vi "write hi scores.vi"(8 "Error In":errorcluster, 10 "file path (dialog if empty)":path, 11 "Score Array In":T1[](array[typedef])) -> (0 "Error Out":errorcluster)   [LabVIEW 2017]
uses:
  controls/scores.ctl
  <vilib>/Utility/file.llb/Write To Spreadsheet File (DBL).vi
  <vilib>/Utility/file.llb/Write To Spreadsheet File (string).vi
panel:
  out "initialized array":string[](array[string])
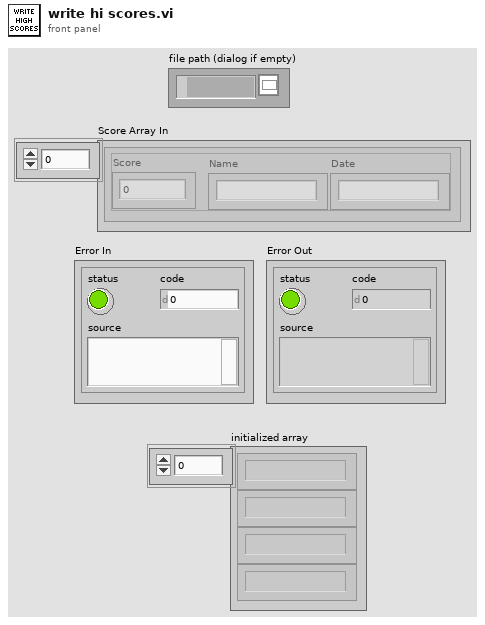
[diagram p1: front panel]
types:
  T1 = typedef "scores.ctl" = cluster{"Score":dbl, "Name":string, "Date":string}
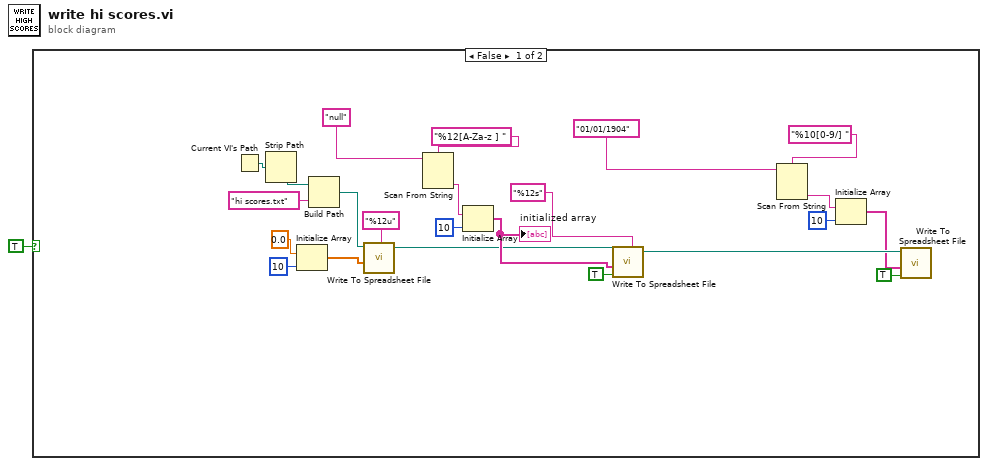
[diagram p0: block diagram]
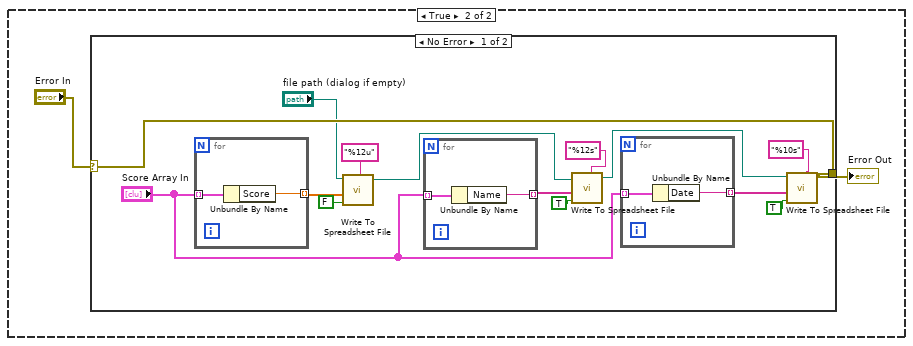
[diagram p2: hidden frame]
diagram:
  n1 = case shown="False" TRUE {
    frame False {
      n2 = Current VI's Path() -> (path=w13:path)
      n3 = Strip Path(path=w13) -> (stripped path=w12:path)  [unwired: 1 out]
      n4 = Initialize Array(0.0 ("element"), 10 ("dimension size")) -> (w15:dbl[])
      n5 = Build Path(base path=w12, name or relative path="hi scores.txt") -> (appended path=w16:path)
      n6 = call-poly <vilib>:"Write To Spreadsheet File.vi"("format (%.3f)"="%12u", "1D data"=w15, "file path (dialog if empty)"=w16) -> ("new file path (Not A Path if cancelled)"=w17:path)  [unwired: 5 in]
      n7 = Scan From String(format string="%12[A-Za-z ] ", input string="null") -> (output 1=w21:string)  [unwired: 3 in, 3 out]
      n8 = Initialize Array(w21, 10 ("dimension size")) -> (w24:string[])
      "initialized array" <- w24
      n9 = call-poly <vilib>:"Write To Spreadsheet File.vi"("format (%s)"="%12s" ("format (%12s)"), "append to file? (new file:F)"=TRUE, "1D data"=w24, "file path (dialog if empty)"=w17) -> ("new file path (Not A Path if cancelled)"=w3:path)  [unwired: 4 in]
      n10 = Scan From String(format string="%10[0-9/] ", input string="01/01/1904") -> (output 1=w6:string)  [unwired: 3 in, 3 out]
      n11 = Initialize Array(w6, 10 ("dimension size")) -> (w2:string[])
      n12 = call-poly <vilib>:"Write To Spreadsheet File.vi"("append to file? (new file:F)"=TRUE, "1D data"=w2, "file path (dialog if empty)"=w3) -> ()  [unwired: 5 in, 1 out]
    }
    frame True {
      n13 = case shown="No Error" "Error In" {
        selector: "Error In" -> [w33 w47]
        tunnel: [w33 w47] -> w25
        frame No Error {
          n14 = for {
            tunnel: "Score Array In" -> [w46] mode=indexing
            tunnel: [w45] -> w37 mode=indexing
            n15 = Unbundle By Name(w46) -> ("Score"=w45:dbl)
          }
          n16 = call-poly <vilib>:"Write To Spreadsheet File.vi"("format (%.3f)"="%12u", "append to file? (new file:F)"=FALSE, "1D data"=w37, "file path (dialog if empty)"="file path (dialog if empty)") -> ("new file path (Not A Path if cancelled)"=w34:path)  [unwired: 4 in]
          n17 = for {
            tunnel: "Score Array In" -> [w44] mode=indexing
            tunnel: [w43] -> w36 mode=indexing
            n18 = Unbundle By Name(w44) -> ("Name"=w43:string)
          }
          n19 = call-poly <vilib>:"Write To Spreadsheet File.vi"("format (%s)"="%12s" ("format (%12s)"), "append to file? (new file:F)"=TRUE, "1D data"=w36, "file path (dialog if empty)"=w34) -> ("new file path (Not A Path if cancelled)"=w30:path)  [unwired: 4 in]
          n20 = for {
            tunnel: [w42] -> w27 mode=indexing
            tunnel: "Score Array In" -> [w41] mode=indexing
            n21 = Unbundle By Name(w41) -> ("Date"=w42:string)
          }
          n22 = call-poly <vilib>:"Write To Spreadsheet File.vi"("format (%s)"="%10s" ("format (%12s)"), "append to file? (new file:F)"=TRUE, "1D data"=w27, "file path (dialog if empty)"=w30) -> ()  [unwired: 4 in, 1 out]
        }
        frame Error {
        }
      }
      "Error Out" <- w25
    }
  }
